vi "HOST_feedback+datapass_accum_8-21-23.vi"() -> ()   [LabVIEW 2020]
uses:
  <vilib>/rvi/interface/nirviMethod/nirviMethod.xnode
  <vilib>/rvi/errors/niLvFpgaMergeErrorWithErrorCode.vi
  <instrlib>/_niInstr/Streaming/v1/Host/niInstr Streaming v1 Host.lvlib
  <vilib>/rvi/interface/nirviReadWriteControl/nirviReadWriteControl.xnode
  <vilib>/rvi/interface/nirviCloseFPGA/nirviCloseFPGA.xnode
  <vilib>/rvi/interface/nirviOpenFPGA/nirviOpenFPGA.xnode
  <vilib>/rvi/interface/Simulation/niFpgaSimulationCallBeginRW.vi
  <vilib>/rvi/errors/niLvFpgaAdjustHostInterfaceError.vi
  NiFpgaLv.dll
  <vilib>/Utility/error.llb/Error Cluster From Error Code.vi
  <vilib>/Utility/file.llb/Write Delimited Spreadsheet (string).vi
  <instrlib>/_niInstr/Streaming/v1/Host/Public/Start Finite Stream.vi
  <instrlib>/_niInstr/Streaming/v1/Host/Public/Wait for Stream.vi
  <instrlib>/_niInstr/Streaming/v1/Host/Public/Start Continuous Stream.vi
  <vilib>/FPGAPlugInAG/Dynamic/niLvFpga_ConfigureFifo_Dynamic.vi
  <vilib>/FPGAPlugInAG/Dynamic/niLvFpga_StartFifo_Dynamic.vi
  <vilib>/FPGAPlugInAG/Dynamic/niLvFpga_ReadFifo_Dynamic.vi
  <vilib>/FPGAPlugInAG/Dynamic/niLvFpga_WriteFifo_Dynamic.vi
  <vilib>/FPGAPlugInAG/Dynamic/niLvFpga_Close_Dynamic.vi
  FPGA Bitfiles/rfsignal_FPGATarget_feedback+datapas_M+I99ZCAYuY.lvbitx
  <vilib>/FPGAPlugInAG/PXIe-7972R/niLvFpga_Open_PXIe-7972R.vi
  <vilib>/rvi/interface/common/dynamic/niFpgaDynamicAddResources.vi
  <vilib>/userdefined/Silver/nirio_resource_slv.ctl
  Controls/Clock Select.ctl
  PID/Typedef/niFpgaPID_ManualControl.ctl
  PID/Typedef/niFpgaPID_PIDGains.ctl
  PID/Typedef/niFpgaPID_OutputRange.ctl
  PID/Typedef/niFpgaPID_SetpointWeightings.ctl
  PID/Typedef/niFpgaPID_PIDActions.ctl
panel:
  in  "Data transfer method":bool
  in  "Downsample":i16
  in  "Signal Delay (us)":i32=5
  out "actions":T1
  out "error":sgl
  out "output":sgl
  out "error 2":sgl
  out "error 3":sgl
  out "output 3":sgl
  out "actions 3":T1
  out "output 2":sgl
  out "actions 2":T1
  in  "Gains Z":T2[](array[typedef]) {"filter coefficient" min=0 max=1; "proportional gain" step=0.125}
  in  "setpoint weighting 3":T3={"proportional weighting (1)"=1.0, "derivative weighting (0)"=0.0} {"derivative weighting (0)" min=0 max=1; "proportional weighting (1)" min=0 max=1}
  in  "output range 3":T4={"output high (Inf)"=inf, "output low (-Inf)"=-inf}
  in  "manual control 3":T5
  in  "reset? (F) 3":bool
  in  "setpoint weighting 2":T3={"proportional weighting (1)"=1.0, "derivative weighting (0)"=0.0} {"derivative weighting (0)" min=0 max=1; "proportional weighting (1)" min=0 max=1}
  in  "output range 2":T4={"output high (Inf)"=inf, "output low (-Inf)"=-inf}
  in  "gains 2":T2 {"filter coefficient" min=0 max=1; "proportional gain" step=0.125}
  in  "manual control 2":T5
  in  "reset? (F) 2":bool
  in  "Feedback scaling z":fxp<+,16,4>
  in  "Feedback scaling x/y":fxp<+,16,4>
  in  "Apply feedback":bool
  in  "Data Trigger Level (V)":dbl
  in  "Record Size":u32=1024
  out "AI":waveform(dbl)[](graph)
  in  "Data Trigger When":enum8{"Trigger Above", "Trigger Below"}(ring)
  in  "Trigger Type":enum8{"Immediate", "Data Trigger", "TRIG input"}(ring)
  in  "Direction switch":bool
  in  "Step gain values":dbl
  in  "?":bool
  in  "% of max CH 1":dbl=85.0
  in  "% of max CH 0":dbl=85.0
  in  "setpoint weighting":T3={"proportional weighting (1)"=1.0, "derivative weighting (0)"=0.0} {"derivative weighting (0)" min=0 max=1; "proportional weighting (1)" min=0 max=1}
  in  "output range":T4={"output high (Inf)"=inf, "output low (-Inf)"=-inf}
  in  "gains":T2 {"filter coefficient" min=0 max=1; "proportional gain" step=0.125}
  in  "manual control":T5
  in  "reset? (F)":bool
  in  "write time ch0":bool
  in  "Record time for power sweep CH0":bool
  in  "Record time for power sweep CH1":bool
  in  "write time ch1":bool
  in  "save path for power calibration (dialog if empty)":path
  out "time check":u16=16
  in  "Cycles per step":u16=30
  in  "Gain Scan Endpoint (CH1)":dbl[](array[numeric])=[100.0, 100.0, 100.0, 100.0, 100.0, 100.0, 100.0, 100.0, 100.0, 100.0, 100.0, 100.0, 100.0, 100.0, 100.0, 100.0, 100.0, 100.0, 100.0, 100.0, 100.0, 100.0, 100.0, 100.0, 100.0, 100.0, 100.0, 100.0, 100.0, 100.0, 100.0, 100.0, 100.0, 100.0, 100.0, 100.0]
  in  "Gain Scan Endpoint (CH0)":dbl[](array[numeric])=[100.0, 100.0, 100.0, 100.0, 100.0, 100.0, 100.0, 100.0, 100.0, 100.0, 100.0, 100.0, 100.0, 100.0, 100.0, 100.0, 100.0, 100.0, 100.0, 100.0, 100.0, 100.0, 100.0, 100.0, 100.0, 100.0, 100.0, 100.0, 100.0, 100.0, 100.0, 100.0, 100.0, 100.0, 100.0, 100.0]
  in  "Scan End Setpoint (CH1)":dbl[](array[numeric])=[23.0, 24.0, 25.0, 26.0, 27.0, 28.0, 23.0, 24.0, 25.0, 26.0, 27.0, 28.0, 23.0, 24.0, 25.0, 26.0, 27.0, 28.0, 23.0, 24.0, 25.0, 26.0, 27.0, 28.0, 23.0, 24.0, 25.0, 26.0, 27.0, 28.0, 23.0, 24.0, 25.0, 26.0, 27.0, 28.0] format="%#_10f"
  in  "Scan CH1":bool
  in  "Scan CH0":bool
  in  "Fq Scan Endpoint (CH0)":dbl[](array[numeric])=[23.0, 23.0, 23.0, 23.0, 23.0, 23.0, 24.0, 24.0, 24.0, 24.0, 24.0, 24.0, 25.0, 25.0, 25.0, 25.0, 25.0, 25.0, 26.0, 26.0, 26.0, 26.0, 26.0, 26.0, 27.0, 27.0, 27.0, 27.0, 27.0, 27.0, 28.0, 28.0, 28.0, 28.0, 28.0, 28.0] format="%#_10f"
  in  "Amp mod on/off":bool[](array[boolean])=[FALSE, FALSE, FALSE, FALSE, FALSE, FALSE, FALSE, FALSE, FALSE]
  in  "Mod Amp (%)":fxp<+,16,1>[](array[numeric])=[1.0, 1.0, 1.0, 1.0, 1.0, 1.0, 1.0, 1.0, 1.0]
  in  "Mod Fq (Hz) 3":dbl[](array[numeric])=[1.0, 1.0, 1.0, 1.0, 1.0, 1.0, 1.0, 1.0, 1.0] format="%#5.5f"
  in  "Wave 2 mod on/off":bool[](array[boolean])=[FALSE, FALSE, FALSE, FALSE, FALSE, FALSE, FALSE, FALSE, FALSE]
  in  "Mod strength (Hz) 2":dbl[](array[numeric])=[100000.0, 100000.0, 100000.0, 100000.0, 100000.0, 100000.0, 100000.0, 100000.0, 100000.0] format="%#_6p"
  in  "Mod Fq (Hz) 2":dbl[](array[numeric])=[1.0, 1.0, 1.0, 1.0, 1.0, 1.0, 1.0, 1.0, 1.0] format="%#5.5f"
  in  "Wave 1 mod on/off":bool[](array[boolean])=[FALSE, FALSE, FALSE, FALSE, FALSE, FALSE, FALSE, FALSE, FALSE]
  in  "Mod strength (Hz)":dbl[](array[numeric])=[100000.0, 100000.0, 100000.0, 100000.0, 100000.0, 100000.0, 100000.0, 100000.0, 100000.0] format="%#_6p"
  in  "Mod Time (Hz)":dbl[](array[numeric])=[1.0, 1.0, 1.0, 1.0, 1.0, 1.0, 1.0, 1.0, 1.0] format="%#5.5p"
  in  "Gain Scan Step Size % (CH1)":dbl=1.0
  in  "Gain Scan Step Size % (CH0)":dbl=1.0
  in  "Fq Scan Step Size MHz (CH1)":dbl=0.1
  in  "Fq Scan Step Size MHz (CH0)":dbl=0.1
  in  "Input pass through\nmode":enum16{"Wire", "Accum-edge"}(ring)
  in  "# of beams":i8=36
  in  "Wave Reader CH 1 (MHz)":dbl[](array[numeric])=[23.0, 24.0, 25.0, 26.0, 27.0, 28.0, 23.0, 24.0, 25.0, 26.0, 27.0, 28.0, 23.0, 24.0, 25.0, 26.0, 27.0, 28.0, 23.0, 24.0, 25.0, 26.0, 27.0, 28.0, 23.0, 24.0, 25.0, 26.0, 27.0, 28.0, 23.0, 24.0, 25.0, 26.0, 27.0, 28.0] format="%#_15f"
  in  "Gain CH 1 (%)":dbl[](array[numeric])=[100.0, 100.0, 100.0, 100.0, 100.0, 100.0, 100.0, 100.0, 100.0, 100.0, 100.0, 100.0, 100.0, 100.0, 100.0, 100.0, 100.0, 100.0, 100.0, 100.0, 100.0, 100.0, 100.0, 100.0, 100.0, 100.0, 100.0, 100.0, 100.0, 100.0, 100.0, 100.0, 100.0, 100.0, 100.0, 100.0]
  in  "Remove transition edges":i32=5
  in  "Time per beam in us":i32=20
  in  "stop":bool
  in  "Gain CH 0 (%)":dbl[](array[numeric])=[100.0, 100.0, 100.0, 100.0, 100.0, 100.0, 100.0, 100.0, 100.0, 100.0, 100.0, 100.0, 100.0, 100.0, 100.0, 100.0, 100.0, 100.0, 100.0, 100.0, 100.0, 100.0, 100.0, 100.0, 100.0, 100.0, 100.0, 100.0, 100.0, 100.0, 100.0, 100.0, 100.0, 100.0, 100.0, 100.0]
  in  "Wave Reader CH 0 (MHz)":dbl[](array[numeric])=[23.0, 23.0, 23.0, 23.0, 23.0, 23.0, 24.0, 24.0, 24.0, 24.0, 24.0, 24.0, 25.0, 25.0, 25.0, 25.0, 25.0, 25.0, 26.0, 26.0, 26.0, 26.0, 26.0, 26.0, 27.0, 27.0, 27.0, 27.0, 27.0, 27.0, 28.0, 28.0, 28.0, 28.0, 28.0, 28.0] format="%#_13f"
  in  "Magnitude Initialization Vpp":dbl[](array[numeric])=[1.0, 1.0] format="%0.2p"
  in  "Frequencies (Hz)":dbl[](array[numeric])=[10000.0, 10000.0] format="%5.0p"
  in  "Signal Type":T6(ring)
  in  "Sampling Info":cluster{"Fs":dbl, "#s":dbl}={"Fs"=163840000.0, "#s"=65536.0} {"Fs" format="%#_5p"}
  out "Error Out":errorcluster
  in  "Update Waveform":bool
  in  "Clock Select":T7 items=["Internal Clock", "Internal Clock w/ Ref via CLK/REF IN", "Internal Clock w/ Ref via Sync Clock", "External Clock via CLK/REF IN"]
  in  "Rate of External Sample Clock (MHz)":u16=100 min=60 max=100 step=1
  in  "RIO Resource":T8="RIO0"
  # "General Feedback Settings"
  # "Time cycle loop processing"
  # "Shared Feedback Controls"
  # "up to 65535"
  # "Don't change"
  # "Waveform Initialization"
  # "Modulation disabled for now while testing FPGA code, too high compiling time for quick turn around"
  # "Controls the Output of the FPGA\nEach row corresponds to one beam created by the AOD\nCH 0 is Output 0 on the FPGA card and controls the () direction on the AOD; CH 1 is Output 1 on the FPGA card and controls the () direction on the AOD\n\nThe  set frequency is the output of the FPGA, this is then mixed with a 50MHz LO to be in the AOD's bandwidth of 75 +- 15MHz\n\nThe gain is the percentage of the 1Vpp initialized voltage to output. It is in percentage and goes from 0 - 100\n\nIt will play the first n rows of tones, \nwhere n is the \"# of beams\" value."
  # "DO NOT CHANGE"
  # "X Feedback"
  # "These allow you to smoothly ramp between frequencies or gain settings for each individual beam.\nThe channels scan independently, but it will simultaneously ramp every fq/gain in the channel to their desired point.\nThey should update to match the main control setting when scanning is not enabled."
  # "Ch 0 Wave Sin Modulation"
  # "Ch 1 Wave Sin Modulation"
  # "Amplitude Sin Modulation"
  # "Do not change these values while waiting for scan"
  # "Main control for the tones played on FPGA analog out 0\nSets the base, static frequency to play"
  # "Main control for the tones played on FPGA analog out 1\nSets the base, static frequency to play"
  # "Ch 0 Output Waveforms"
  # "Ch 1 Output Waveforms"
  # "Y Feedback"
  # "Ch0"
  # "Ch1"
  # "Modulates the output frequencies of CH 0 in a sine wave pattern\n\nMod time: Sets how fast the modulation goes\n     (e.g. 1 Hz means it will go through a full cycle in 1 second)\n\nMod strength: Sets the amplitude of the modulation\n     (e.g. 100kHz means that the frequency will go between \n      set frequency + 100kHz and set frequency - 100kHz)"
  # "Modulates the output frequencies of CH 1 in a sine wave pattern\n\nMod time: Sets how fast the modulation goes\n     (e.g. 1 Hz means it will go through a full cycle in 1 second)\n\nMod strength: Sets the amplitude of the modulation\n     (e.g. 100kHz means that the frequency will go between \n      set frequency + 100kHz and set frequency - 100kHz)"
  # "Modulates the output amplitude of CH 0 in a sine wave pattern\n\nMod time: Sets how fast the modulation goes\n     (e.g. 1 Hz means it will go through a full cycle in 1 second)\n\nMod strength: Sets the amplitude of the modulation\n     (e.g. 5% means that the amplitude will go between \n      set amp + 5%  and set amp  - 5%)"
  # "Z\nFeedback"
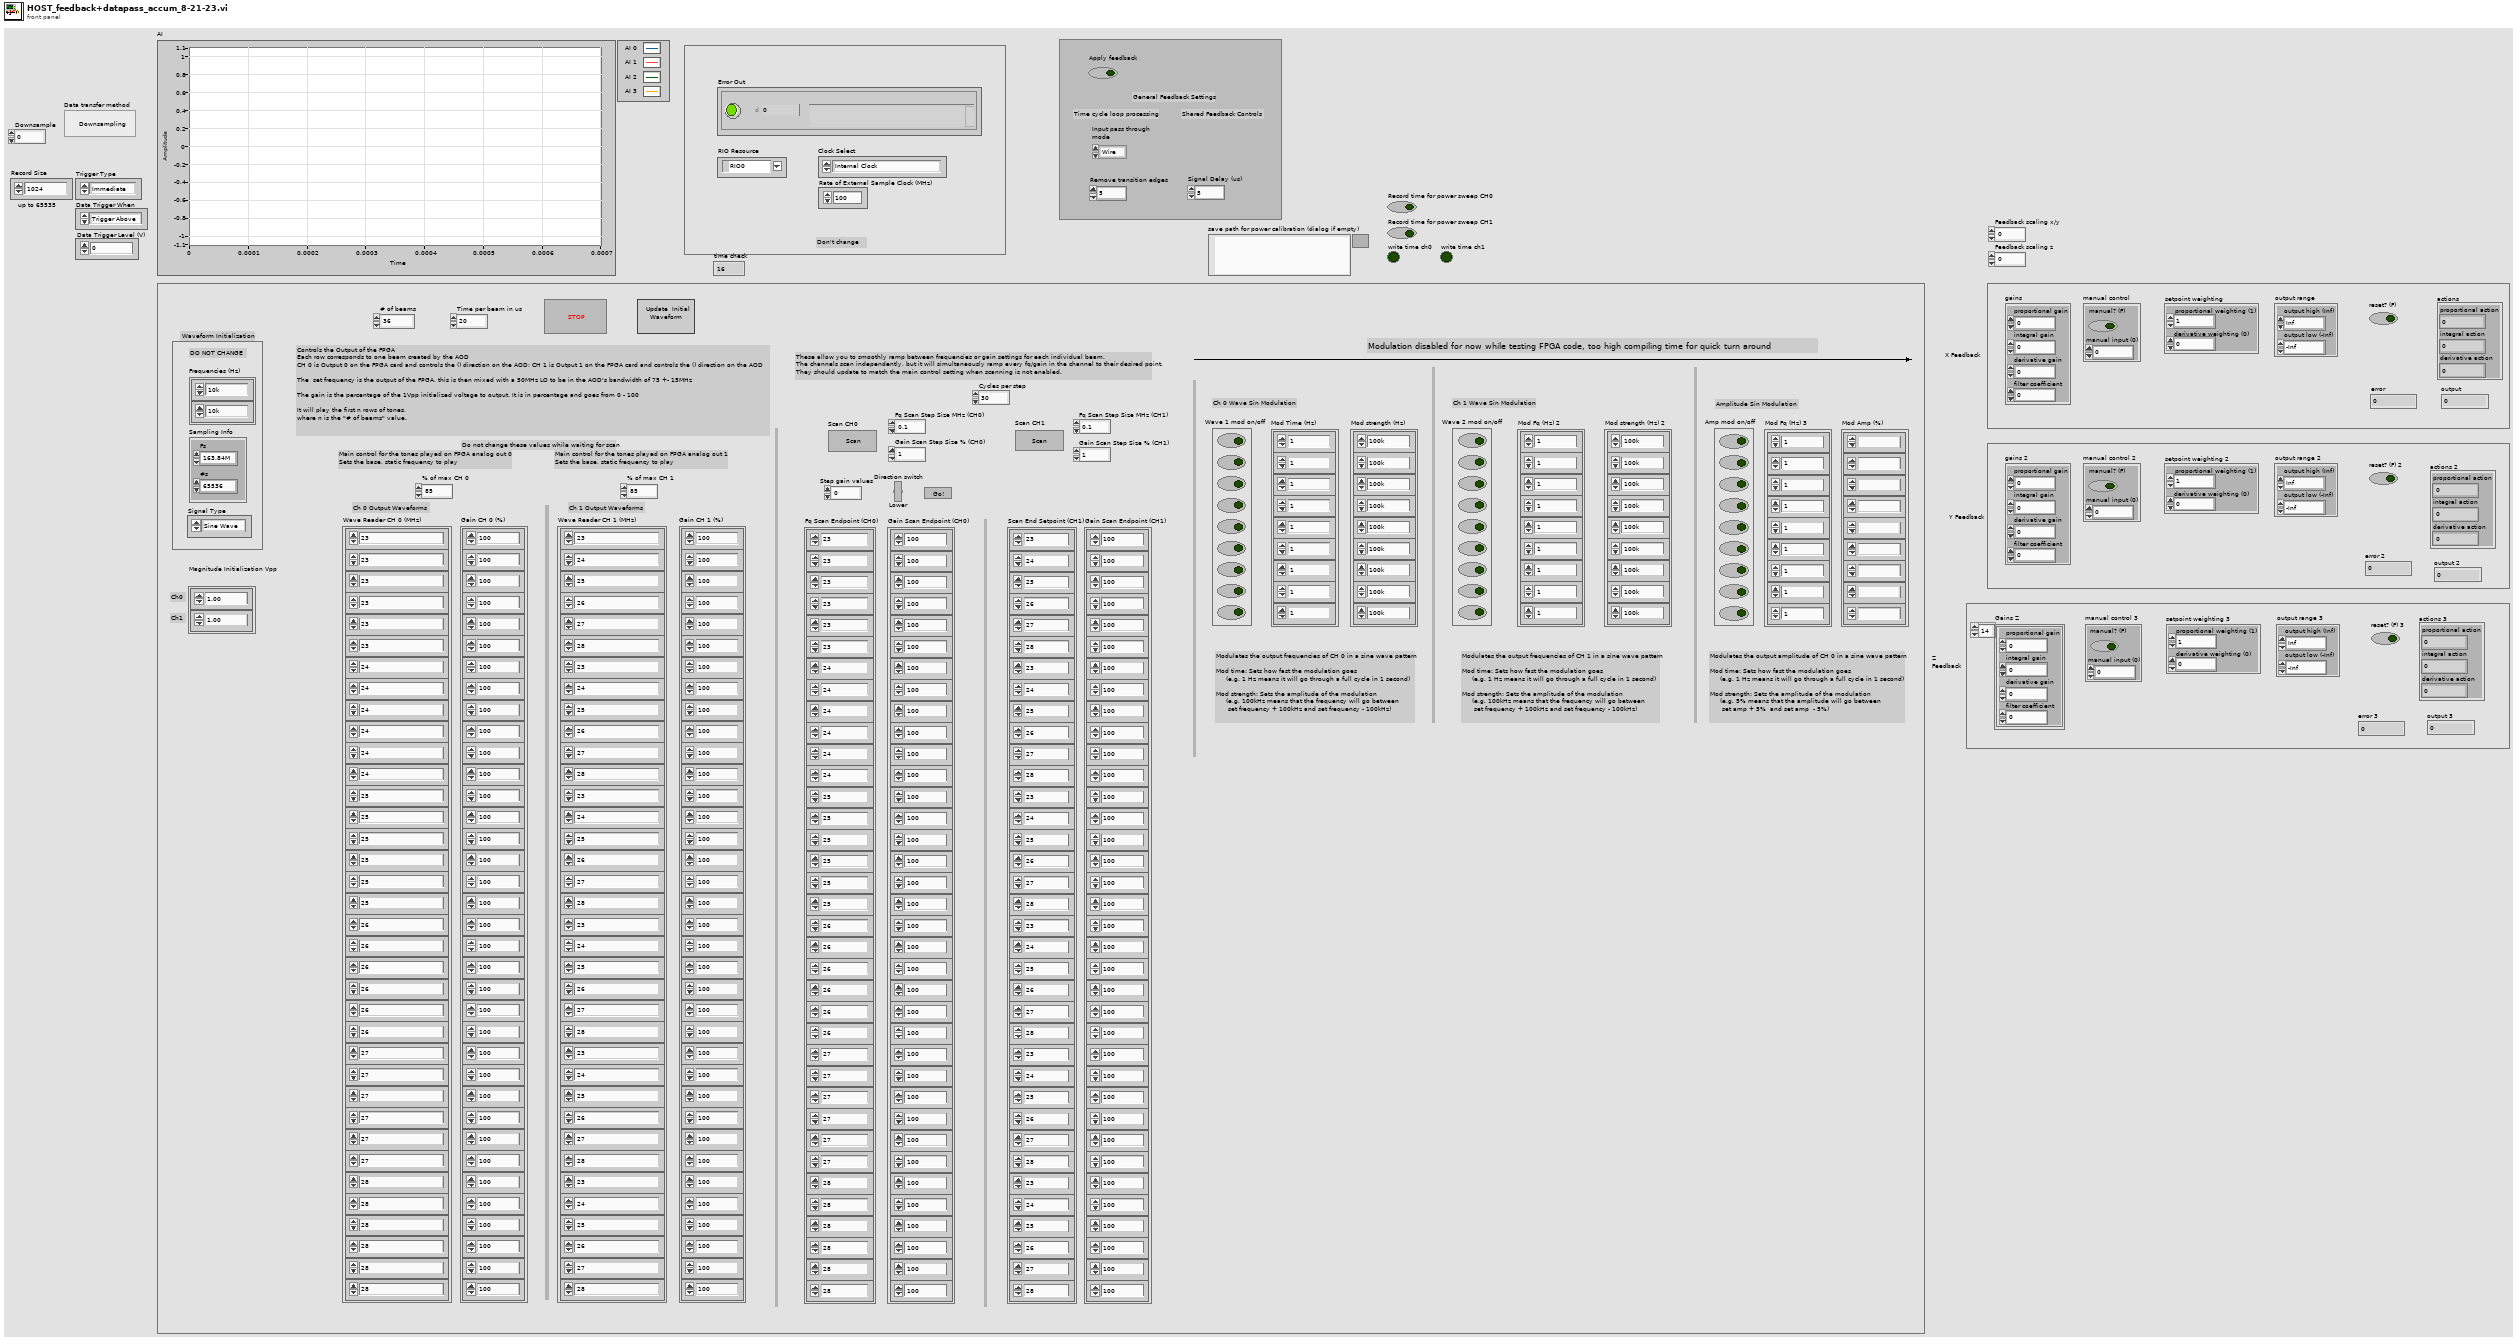
[diagram p1: front panel]
types:
  T1 = typedef "niFpgaPID_PIDActions.ctl" = cluster{"proportional action":sgl, "integral action":sgl, "derivative action":sgl}
  T2 = typedef "niFpgaPID_PIDGains.ctl" = cluster{"proportional gain":sgl, "integral gain":sgl, "derivative gain":sgl, "filter coefficient":sgl}
  T3 = typedef "niFpgaPID_SetpointWeightings.ctl" = cluster{"proportional weighting (1)":sgl, "derivative weighting (0)":sgl}
  T4 = typedef "niFpgaPID_OutputRange.ctl" = cluster{"output high (Inf)":sgl, "output low (-Inf)":sgl}
  T5 = typedef "niFpgaPID_ManualControl.ctl" = cluster{"manual? (F)":bool, "manual input (0)":sgl}
  T6 = enum16{"Sine Wave", "Triangle Wave", "Square Wave", "Sawtooth Wave"}
  T7 = typedef "Clock Select.ctl" = u16
  T8 = typedef "nirio_resource_slv.ctl" = tag
  T9 = cluster{"proportional action":sgl, "integral action":sgl, "derivative action":sgl}
  T10 = cluster{"level":i16, "trigger when":enum8{"Trigger Above", "Trigger Below"}}
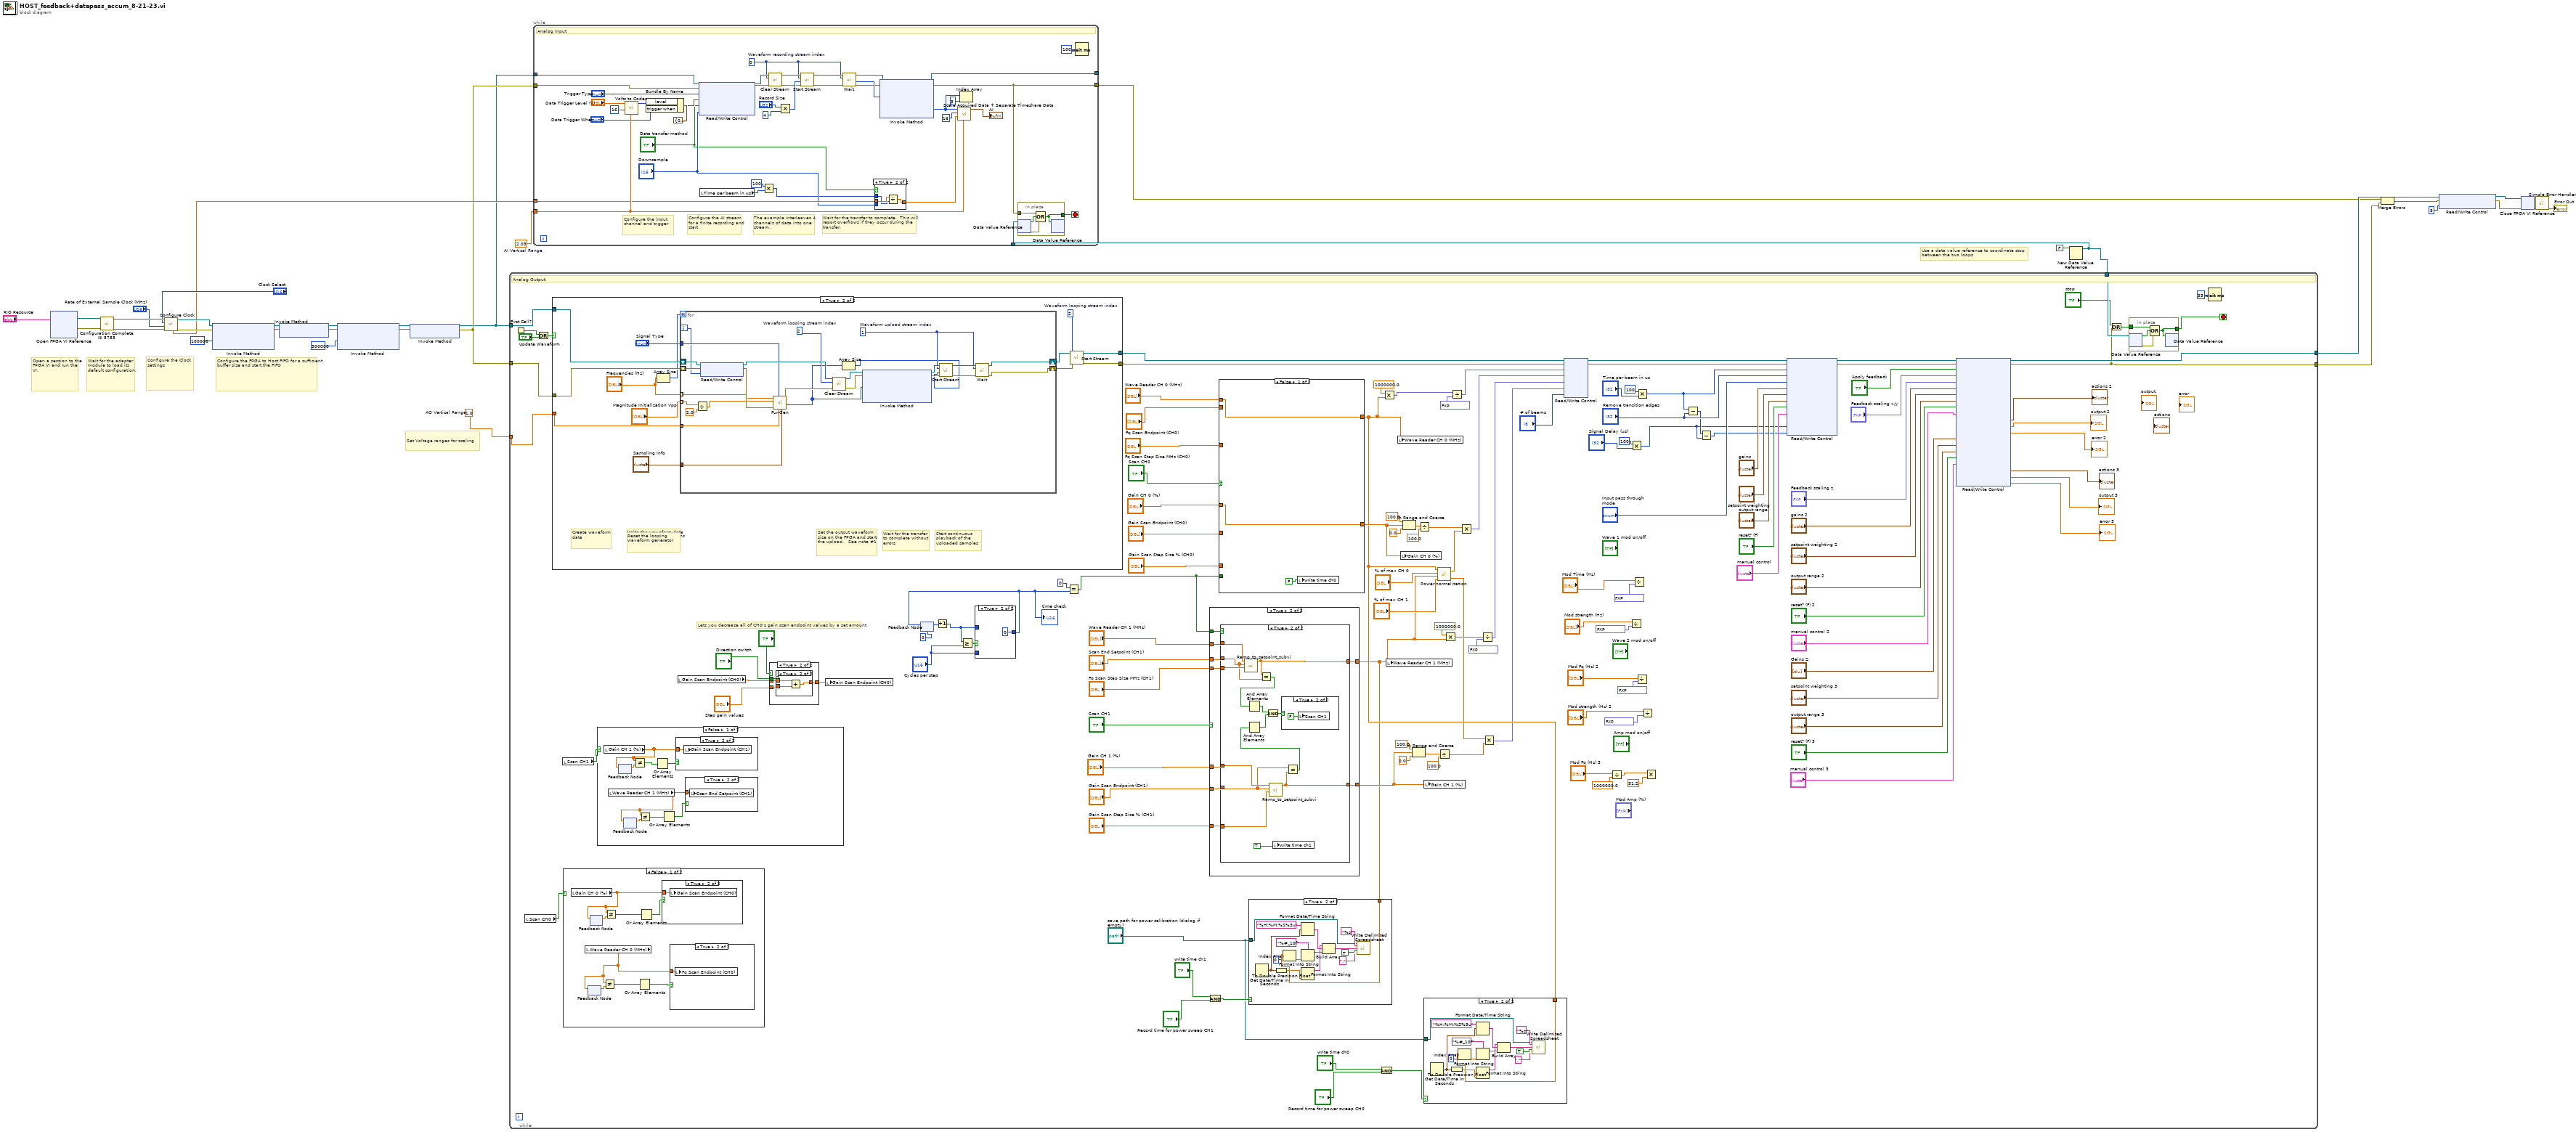
[diagram p0: block diagram]
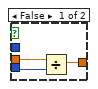
[diagram p2: hidden frame]
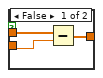
[diagram p4: hidden frame]
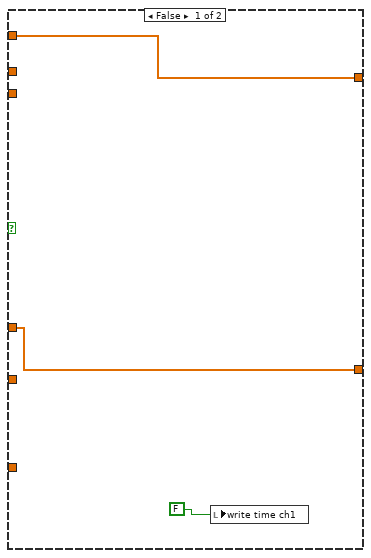
[diagram p7: hidden frame]
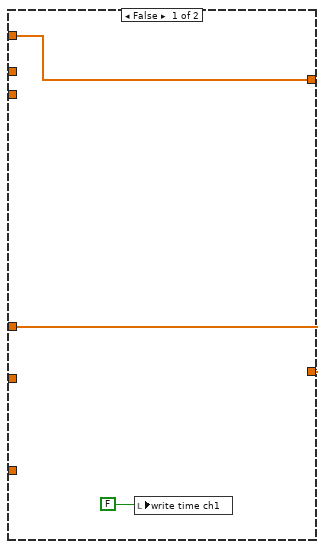
[diagram p8: hidden frame]
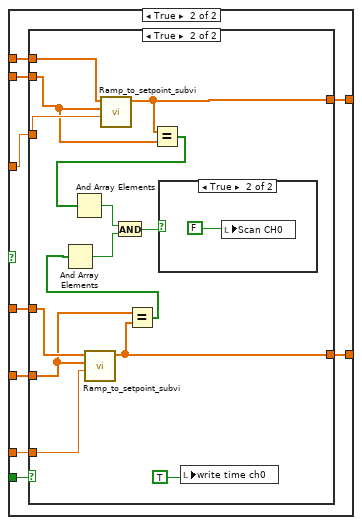
[diagram p10: hidden frame]
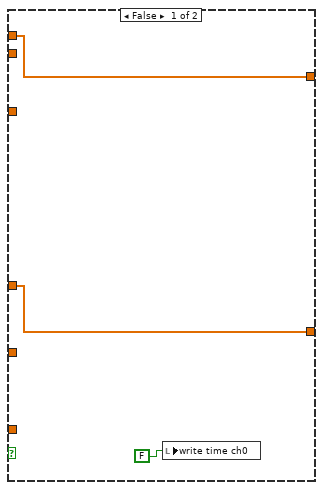
[diagram p11: hidden frame]
diagram:
  w13 = 2.03  # AI Vertical Range
  w21 = 1.0  # AO Vertical Range
  # "Use a data value reference to coordinate stop between the two loops"
  # "Set Voltage ranges for scaling"
  # "Configure the Clock settings"
  # "Configure the FPGA to Host FIFO for a sufficient buffer size and start the FIFO"
  # "Wait for the adapter module to load its default configuration."
  # "Open a session to the FPGA VI and run the VI."
  n1 = xnode "Open FPGA VI Reference"("resource name"="RIO Resource") -> ("FPGA VI Reference Out"=w19:refnum<k20>, "error out"=w18:errorcluster)  [unwired: 1 in]
  n2 = call "Configuration Complete NI 5783.vi"("error in"=w18, "FPGA VI Reference In"=w19) -> ("error out"=w29:errorcluster, "FPGA VI Reference Out"=w30:refnum<k20>)  [unwired: 7 in, 1 out]
  n3 = call "Configure Clock.vi"("error in (no error)"=w29, "Rate of External Sample Clock (MHz)"="Rate of External Sample Clock (MHz)", "Clock Select"="Clock Select", "FPGA VI Reference In"=w30) -> ("error out"=w27:errorcluster, "FPGA VI Reference Out"=w28:refnum<k20>, "Sampling Rate"=w12:dbl)  [unwired: 3 in, 2 out]
  n4 = xnode "Invoke Method"("FPGA VI Reference In"=w28, "error in"=w27, "Requested Depth"=u32 100000) -> ("FPGA VI Reference Out"=w33:refnum<k20>, "error out"=w32:errorcluster)  [unwired: 1 out]
  n5 = xnode "Invoke Method"("FPGA VI Reference In"=w33, "error in"=w32) -> ("FPGA VI Reference Out"=w4:refnum<k20>, "error out"=w7:errorcluster)
  n6 = xnode "Invoke Method"("FPGA VI Reference In"=w4, "error in"=w7, "Requested Depth"=u32 300000) -> ("FPGA VI Reference Out"=w3:refnum<k20>, "error out"=w6:errorcluster)  [unwired: 1 out]
  n7 = xnode "Invoke Method"("FPGA VI Reference In"=w3, "error in"=w6) -> ("FPGA VI Reference Out"=w2:refnum<k20>, "error out"=w5:errorcluster)
  n8 = New Data Value Reference(data value=FALSE ("Stopped")) -> (data value reference=w10:refnum<data-value>)  [unwired: 1 in, 1 out]
  n9 = while {
    tunnel: w5 -> [w157]
    tunnel: w2 -> [w163]
    tunnel: [w61] -> w17
    tunnel: w10 -> [w158]
    tunnel: w21 -> [w156]
    tunnel: [w59] -> w8
    stop <- w66 stop-if-true
    # "Lets you decrease all of CH0's gain scan endpoint values by a set amount"
    # "Analog Output"
    n10 = First Call?() -> (First Call?: T/F=w159:bool)
    n11 = local read "Scan CH0"() -> (w109:bool)
    n12 = Or(x=w159, y="Update Waveform") -> (x .or. y?=w160:bool)
    n13 = case shown="True" w160 {
      tunnel: [w292 w305] -> w155
      tunnel: [w291 w304] -> w154
      tunnel: w163 -> [w292 w302]
      tunnel: w157 -> [w291 w301]
      tunnel: w156 -> [_ w303]
      frame False {
      }
      frame True {
        w300 = 2  # Waveform looping stream index
        # "Loop over the waveforms to combine"
        # "Reset the looping waveform generator"
        # "Start continuous playback of the uploaded samples"
        # "Wait for the transfer to complete without errors"
        # "Set the output waveform size on the FPGA and start the upload.   See note #1"
        # "Write the waveform data to the FPGA for generation"
        # "Create waveform data"
        n14 = Array Size(array="Frequencies (Hz)") -> (size(s)=w295:i32)
        n15 = for {
          N: w295 -> [_]
          tunnel: w303 -> [w320]
          shift-right: [w314] -> w299
          shift-left: w302 -> [w319]
          shift-right: [w313] -> w298
          shift-left: w301 -> [w317]
          tunnel: "Frequencies (Hz)" -> [w312] mode=indexing
          tunnel: "Magnitude Initialization Vpp" -> [w308] mode=indexing
          tunnel: "Sampling Info" -> [w311]
          tunnel: "Signal Type" -> [w310]
          i -> [w309]
          w321 = 2  # Waveform looping stream index
          w326 = 1  # Waveform upload stream index
          n16 = Divide(x=w308, y=2.0) -> (x/y=w307:dbl)
          n17 = xnode "Read/Write Control"("FPGA VI Reference In"=w319, "error in"=w317, "Upload selector"=w309) -> ("FPGA VI Reference Out"=w318:refnum<k20>, "error out"=w316:errorcluster)
          n18 = call "FunGen.vi"("sampling info"=w311, "range (Vpp)"=w320, "signal type"=w310, "error in (no error)"=w316, "amplitude"=w307, "frequency"=w312) -> ("error out"=w322:errorcluster, "Waveform Data"=w315:i16[])  [unwired: 2 in, 2 out]
          n19 = call <instrlib>:"Clear Stream.vi"("error in (no error)"=w322, "stream index"=w321, "refnum in"=w318) -> ("error out"=w324:errorcluster, "refnum out"=w325:refnum<k20>)  [unwired: 7 in]
          n20 = Array Size(array=w315) -> (size(s)=w323:i32)
          n21 = xnode "Invoke Method"("FPGA VI Reference In"=w325, "error in"=w324, "Data"=w315) -> ("FPGA VI Reference Out"=w330:refnum<k20>, "error out"=w329:errorcluster)  [unwired: 1 in, 1 out]
          n22 = call-poly <instrlib>:"Start Stream.vi"("error in (no error)"=w329, "num samples"=w323, "stream index"=w326, "refnum in"=w330) -> ("error out"=w327:errorcluster, "refnum out"=w328:refnum<k20>)  [unwired: 6 in]
          n23 = call-poly <instrlib>:"Wait.vi"("error in (no error)"=w327, "stream index"=w326, "refnum in"=w328) -> ("error out"=w313:errorcluster, "refnum out"=w314:refnum<k20>)  [unwired: 5 in, 2 out]
        }
        n24 = call-poly <instrlib>:"Start Stream.vi"("error in (no error)"=w298, "stream index"=w300, "refnum in"=w299) -> ("error out"=w304:errorcluster, "refnum out"=w305:refnum<k20>)  [unwired: 7 in]
      }
    }
    n25 = local read "Scan CH1"() -> (w110:bool)
    n26 = case shown="False" w109 {
      frame False {
        n27 = local read "Gain CH 0 (%)"() -> (w267:dbl[])
        n28 = local read "Wave Reader CH 0 (MHz)"() -> (w274:dbl[])
        n29 = feedback-in #1(w274) -> ()
        n30 = feedback #1() -> (w273:dbl[])  [unwired: 1 in]
        n31 = feedback #2() -> (w270:dbl[])  [unwired: 1 in]
        n32 = feedback-in #2(w267) -> ()
        n33 = Not Equal?(x=w274, y=w273) -> (x != y?=w272:bool[])
        n34 = Not Equal?(x=w267, y=w270) -> (x != y?=w269:bool[])
        n35 = Or Array Elements(Boolean array=w272) -> (logical OR=w271:bool)
        n36 = Or Array Elements(Boolean array=w269) -> (logical OR=w268:bool)
        n37 = case shown="True" w268 {
          tunnel: w267 -> [_ w275]
          frame False {
          }
          frame True {
            n38 = local write "Gain Scan Endpoint (CH0)"(w275) -> ()
          }
        }
        n39 = case shown="True" w271 {
          tunnel: w274 -> [_ w276]
          frame False {
          }
          frame True {
            n40 = local write "Fq Scan Endpoint (CH0)"(w276) -> ()
          }
        }
      }
      frame True {
      }
    }
    n41 = case shown="False" w110 {
      frame False {
        n42 = local read "Gain CH 1 (%)"() -> (w277:dbl[])
        n43 = local read "Wave Reader CH 1 (MHz)"() -> (w281:dbl[])
        n44 = feedback #3() -> (w280:dbl[])  [unwired: 1 in]
        n45 = feedback-in #3(w277) -> ()
        n46 = feedback #4() -> (w284:dbl[])  [unwired: 1 in]
        n47 = feedback-in #4(w281) -> ()
        n48 = Not Equal?(x=w277, y=w280) -> (x != y?=w279:bool[])
        n49 = Not Equal?(x=w281, y=w284) -> (x != y?=w283:bool[])
        n50 = Or Array Elements(Boolean array=w279) -> (logical OR=w278:bool)
        n51 = Or Array Elements(Boolean array=w283) -> (logical OR=w282:bool)
        n52 = case shown="True" w278 {
          tunnel: w277 -> [_ w285]
          frame False {
          }
          frame True {
            n53 = local write "Gain Scan Endpoint (CH1)"(w285) -> ()
          }
        }
        n54 = case shown="True" w282 {
          tunnel: w281 -> [_ w286]
          frame False {
          }
          frame True {
            n55 = local write "Scan End Setpoint (CH1)"(w286) -> ()
          }
        }
      }
      frame True {
      }
    }
    n56 = local read "Gain Scan Endpoint (CH0)"() -> (w68:dbl[])
    n57 = case shown="True" "?" {
      tunnel: w68 -> [w164 w167]
      tunnel: [w164 w168] -> w69
      tunnel: "Step gain values" -> [_ w166]
      tunnel: "Direction switch" -> [_ w165]
      frame False {
      }
      frame True {
        n58 = case shown="True" w165 {
          tunnel: [w171 w173] -> w168
          tunnel: w167 -> [w170 w172]
          tunnel: w166 -> [w169 w174]
          frame False {
            n59 = Subtract(x=w170, y=w169) -> (x-y=w171:dbl[])
          }
          frame True {
            n60 = Add(x=w172, y=w174) -> (x+y=w173:dbl[])
          }
        }
      }
    }
    n61 = local write "Gain Scan Endpoint (CH0)"(w69) -> ()
    n62 = feedback #5(u16 0) -> (w105:u16)
    n63 = Increment(x=w105) -> (x+1=w103:u16)
    n64 = Greater Or Equal?(x=w103, y="Cycles per step") -> (x >= y?=w104:bool)
    n65 = case shown="True" w104 {
      tunnel: w103 -> [w265 _]
      tunnel: "Cycles per step" -> [_ _]
      tunnel: [w265 u16 0] -> w98
      frame False {
      }
      frame True {
      }
    }
    "time check" <- w98
    n66 = feedback-in #5(w98) -> ()
    n67 = Equal?(x=u16 0, y=w98) -> (x = y?=w99:bool)
    n68 = And(x="write time ch1", y="Record time for power sweep CH1") -> (x .and. y?=w97:bool)
    n69 = case shown="True" "Scan CH1" {
      tunnel: "Fq Scan Step Size MHz (CH1)" -> [_ w216]
      tunnel: [w207 w215] -> w77
      tunnel: "Wave Reader CH 1 (MHz)" -> [w207 w214]
      tunnel: "Scan End Setpoint (CH1)" -> [_ w213]
      tunnel: "Gain Scan Step Size % (CH1)" -> [_ w212]
      tunnel: "Gain CH 1 (%)" -> [w206 w211]
      tunnel: "Gain Scan Endpoint (CH1)" -> [_ w210]
      tunnel: [w206 w209] -> w111
      tunnel: w99 -> [_ w208]
      frame False {
        n70 = local write "write time ch1"(FALSE) -> ()
      }
      frame True {
        n71 = case shown="True" w208 {
          tunnel: w214 -> [w219 w233]
          tunnel: w213 -> [_ w231]
          tunnel: w216 -> [_ w232]
          tunnel: [w219 w230] -> w215
          tunnel: w211 -> [w218 w228]
          tunnel: w210 -> [_ w227]
          tunnel: w212 -> [_ w226]
          tunnel: [w218 w221] -> w209
          frame False {
            n72 = local write "write time ch1"(FALSE) -> ()
          }
          frame True {
            n73 = call "Ramp_to_setpoint_subvi.vi"("Numeric"=w232, "Scan to Fq (CH0)"=w231, "Wave Reader CH 0 (Y)"=w233) -> ("Array"=w230:dbl[])  [unwired: 8 in]
            n74 = Equal?(x=w230, y=w231) -> (x = y?=w229:bool[])
            n75 = And Array Elements(Boolean array=w229) -> (logical AND=w223:bool)
            n76 = call "Ramp_to_setpoint_subvi.vi"("Numeric"=w226, "Scan to Fq (CH0)"=w227, "Wave Reader CH 0 (Y)"=w228) -> ("Array"=w221:dbl[])  [unwired: 8 in]
            n77 = local write "write time ch1"(TRUE) -> ()
            n78 = Equal?(x=w227, y=w221) -> (x = y?=w222:bool[])
            n79 = And Array Elements(Boolean array=w222) -> (logical AND=w224:bool)
            n80 = And(x=w223, y=w224) -> (x .and. y?=w225:bool)
            n81 = case shown="True" w225 {
              frame False {
              }
              frame True {
                n82 = local write "Scan CH1"(FALSE) -> ()
              }
            }
          }
        }
      }
    }
    n83 = case shown="False" "Scan CH0" {
      tunnel: "Fq Scan Step Size MHz (CH0)" -> [_ w246]
      tunnel: "Wave Reader CH 0 (MHz)" -> [w237 w245]
      tunnel: "Fq Scan Endpoint (CH0)" -> [_ w244]
      tunnel: [w237 w243] -> w78
      tunnel: "Gain CH 0 (%)" -> [w236 w242]
      tunnel: "Gain Scan Endpoint (CH0)" -> [_ w241]
      tunnel: [w236 w240] -> w119
      tunnel: "Gain Scan Step Size % (CH0)" -> [_ w239]
      tunnel: w99 -> [_ w238]
      frame False {
        n84 = local write "write time ch0"(FALSE) -> ()
      }
      frame True {
        n85 = case shown="True" w238 {
          tunnel: w245 -> [w249 w263]
          tunnel: w244 -> [_ w261]
          tunnel: w246 -> [_ w262]
          tunnel: [w249 w260] -> w243
          tunnel: w242 -> [w248 w258]
          tunnel: w241 -> [_ w255]
          tunnel: w239 -> [_ w257]
          tunnel: [w248 w256] -> w240
          frame False {
            n86 = local write "write time ch0"(FALSE) -> ()
          }
          frame True {
            n87 = call "Ramp_to_setpoint_subvi.vi"("Numeric"=w257, "Scan to Fq (CH0)"=w255, "Wave Reader CH 0 (Y)"=w258) -> ("Array"=w256:dbl[])  [unwired: 8 in]
            n88 = call "Ramp_to_setpoint_subvi.vi"("Numeric"=w262, "Scan to Fq (CH0)"=w261, "Wave Reader CH 0 (Y)"=w263) -> ("Array"=w260:dbl[])  [unwired: 8 in]
            n89 = Equal?(x=w255, y=w256) -> (x = y?=w254:bool[])
            n90 = And Array Elements(Boolean array=w254) -> (logical AND=w251:bool)
            n91 = Equal?(x=w260, y=w261) -> (x = y?=w259:bool[])
            n92 = And Array Elements(Boolean array=w259) -> (logical AND=w252:bool)
            n93 = And(x=w252, y=w251) -> (x .and. y?=w253:bool)
            n94 = case shown="True" w253 {
              frame False {
              }
              frame True {
                n95 = local write "Scan CH0"(FALSE) -> ()
              }
            }
            n96 = local write "write time ch0"(TRUE) -> ()
          }
        }
      }
    }
    n97 = case shown="True" w97 {
      tunnel: w77 -> [_ w197]
      tunnel: "save path for power calibration (dialog if empty)" -> [_ w190]
      frame False {
      }
      frame True {
        n98 = Get Date/Time In Seconds() -> (seconds since 1Jan1904=w193:timestamp)
        n99 = To Double Precision Float(number=w193) -> (double precision float=w192:dbl)
        n100 = Index Array(array=w197, index=0) -> (element=w195:dbl)
        n101 = Format Date/Time String(time format string (%c)="%H:%M:%S%3u", seconds (now)=w193) -> (date/time string=w200:string)  [unwired: 1 in]
        n102 = Format Into String(format string="%#_10f", w195) -> (resulting string=w199:string)  [unwired: 2 in, 1 out]
        n103 = Format Into String(w192) -> (resulting string=w191:string)  [unwired: 3 in, 1 out]
        n104 = Build Array(w191, w200, w199) -> (w194:string[])
        n105 = call-poly <vilib>:"Write Delimited Spreadsheet.vi"("file path (dialog if empty)"=w190, "format (%s)"="%s" ("format (%.3f)"), "1D data"=w194, "append to file? (new file:F)"=TRUE, "delimiter (\\t)"="," ("delimiter (\\t)")) -> ()  [unwired: 9 in, 2 out]
      }
    }
    n106 = And(x="write time ch0", y="Record time for power sweep CH0") -> (x .and. y?=w93:bool)
    n107 = Multiply(x=1000000.0, y=w78) -> (x*y=w131:fxp<+/-,64,32>[])
    n108 = local write "Wave Reader CH 1 (MHz)"(w77) -> ()
    n109 = local write "Wave Reader CH 0 (MHz)"(w78) -> ()
    n110 = local write "Gain CH 0 (%)"(w119) -> ()
    n111 = In Range and Coerce(upper limit=100.0, x=w119, lower limit=0.0) -> (coerced(x)=w122:dbl[])  [unwired: 1 out]
    n112 = In Range and Coerce(upper limit=100.0, x=w111, lower limit=0.0) -> (coerced(x)=w117:dbl[])  [unwired: 1 out]
    n113 = Divide(x=w122, y=100.0) -> (x/y=w82:dbl[])
    n114 = local write "Gain CH 1 (%)"(w111) -> ()
    n115 = case shown="True" w93 {
      tunnel: w78 -> [_ w182]
      tunnel: "save path for power calibration (dialog if empty)" -> [_ w175]
      frame False {
      }
      frame True {
        n116 = Get Date/Time In Seconds() -> (seconds since 1Jan1904=w178:timestamp)
        n117 = To Double Precision Float(number=w178) -> (double precision float=w177:dbl)
        n118 = Index Array(array=w182, index=0) -> (element=w180:dbl)
        n119 = Format Date/Time String(time format string (%c)="%H:%M:%S%3u", seconds (now)=w178) -> (date/time string=w185:string)  [unwired: 1 in]
        n120 = Format Into String(format string="%#_10f", w180) -> (resulting string=w184:string)  [unwired: 2 in, 1 out]
        n121 = Format Into String(w177) -> (resulting string=w176:string)  [unwired: 3 in, 1 out]
        n122 = Build Array(w176, w185, w184) -> (w179:string[])
        n123 = call-poly <vilib>:"Write Delimited Spreadsheet.vi"("file path (dialog if empty)"=w175, "format (%s)"="%s" ("format (%.3f)"), "1D data"=w179, "append to file? (new file:F)"=TRUE, "delimiter (\\t)"="," ("delimiter (\\t)")) -> ()  [unwired: 9 in, 2 out]
      }
    }
    n124 = call "Power normalization.vi"("% of max CH 1"="% of max CH 1", "CH 1 frequency"=w77, "% of max CH 0"="% of max CH 0", "CH 0 frequency"=w78) -> ("Normalized CH1"=w74:dbl[], "Normalized CH 0"=w79:dbl[])
    n125 = Divide(x=w117, y=100.0) -> (x/y=w75:dbl[])
    n126 = Multiply(x=1000000.0, y=w77) -> (x*y=w128:fxp<+/-,64,32>[])
    n127 = Divide(x=w131, y=fxp<+,32,16> 6103.515625) -> (x/y=w90:fxp<+,33,16>[])
    n128 = Multiply(x=w82, y=w79) -> (x*y=w83:fxp<+,32,4>[])
    n129 = Divide(x=w128, y=fxp<+,32,16> 6103.515625) -> (x/y=w89:fxp<+,33,16>[])
    n130 = Multiply(x=w74, y=w75) -> (x*y=w76:fxp<+,32,4>[])
    n131 = xnode "Read/Write Control"("FPGA VI Reference In"=w155, "error in"=w154, "Wave 1"=w90, "Amp 1"=w83, "Wave 2"=w89, "Amp 2"=w76, "Size"="# of beams") -> ("FPGA VI Reference Out"=w152:refnum<k20>, "error out"=w151:errorcluster)
    n132 = Divide(x="Mod Fq (Hz) 3", y=1000000.0) -> (x/y=w141:dbl[])
    n133 = Divide(x="Mod strength (Hz)", y=fxp<+,32,16> 6103.515625) -> ()  [unwired: 1 out]
    n134 = Multiply(x=100, y="Signal Delay (us)") -> (x*y=w35:i32)
    n135 = Divide(x="Mod Time (Hz)", y=fxp<+,32,16> 6103.515625) -> ()  [unwired: 1 out]
    n136 = Divide(x="Mod Fq (Hz) 2", y=fxp<+,32,16> 6103.515625) -> ()  [unwired: 1 out]
    n137 = Multiply(x=100, y="Time per beam in us") -> (x*y=w38:i32)
    n138 = Divide(x="Mod strength (Hz) 2", y=fxp<+,32,16> 6103.515625) -> ()  [unwired: 1 out]
    n139 = Multiply(x=w141, y=51.2) -> ()  [unwired: 1 out]
    n140 = Subtract(x=w38, y="Remove transition edges") -> (x-y=w36:i32)
    n141 = Subtract(x=w36, y=w35) -> (x-y=w34:i32)
    n142 = xnode "Read/Write Control"("FPGA VI Reference In"=w152, "error in"=w151, "Timeshare"=w38, "Edge size"="Remove transition edges", "Pass selector"="Input pass through\nmode", "gains"="gains", "setpoint weighting"="setpoint weighting", "output range"="output range", "reset? (F)"="reset? (F)", "manual control"="manual control", "Signal Delay"=w35, "Data collection size"=w34) -> ("FPGA VI Reference Out"=w62:refnum<k20>, "error out"=w63:errorcluster)  [unwired: 1 in]
    n143 = xnode "Read/Write Control"("FPGA VI Reference In"=w62, "error in"=w63, "Apply feedback"="Apply feedback", "Feedback scaling x/y"="Feedback scaling x/y", "Feedback scaling z"="Feedback scaling z", "gains 2"="gains 2", "setpoint weighting 2"="setpoint weighting 2", "output range 2"="output range 2", "reset? (F) 2"="reset? (F) 2", "manual control 2"="manual control 2", "Gains Z"="Gains Z", "setpoint weighting 3"="setpoint weighting 3", "output range 3"="output range 3", "reset? (F) 3"="reset? (F) 3", "manual control 3"="manual control 3") -> ("FPGA VI Reference Out"=w61:refnum<k20>, "error out"=w59:errorcluster, "actions 2"=→"actions 2":T9, "output 2"=→"output 2":sgl, "error 2"=→"error 2":sgl, "actions 3"=→"actions 3":T9, "output 3"=→"output 3":sgl, "error 3"=→"error 3":sgl)
    n144 = Or(x="stop", y=w59) -> (x .or. y?=w65:bool)
    n145 = in-place {
      in-place-border: [w289] -> w66
      in-place-border: w65 -> [w287]
      n146 = in-place-dvr #6(w158) -> (w290:bool, w288:errorcluster)
      n147 = Compound Arithmetic op=OR(w287, w290, w288) -> (w289:bool)
      n148 = in-place-dvr #6(w289) -> ()  [unwired: 2 out]
    }
    n149 = Wait (ms)(milliseconds to wait=u32 33) -> ()  [unwired: 1 out]
  }
  n150 = while {
    tunnel: [w368] -> _
    tunnel: w2 -> [w367]
    tunnel: w13 -> [w351]
    tunnel: w10 -> [w364]
    tunnel: w5 -> [w366]
    tunnel: [w355] -> w9
    tunnel: w12 -> [w339]
    stop <- w365 stop-if-true
    w343 = 0  # Waveform recording stream index
    # "The example interleaves 4 channels of data into one stream."
    # "Wait for the transfer to complete.  This will report overflows if they occur during the transfer."
    # "Configure the AI stream for a finite recording and start"
    # "Configure the input channel and trigger"
    # "Analog Input"
    n151 = call "Volts to Codes.vi"("range (Vpp)"=w351, "Number of Bits"=i16 16, "Volts In"="Data Trigger Level (V)") -> ("ADC Codes Out"=w352:i16)  [unwired: 8 in]
    n152 = Bundle By Name(cluster=T10 {"level"=0, "trigger when"=enum."Trigger Above"} ("Trigger Configuration"), "level"=w352, "trigger when"="Data Trigger When") -> (w342:T10)
    n153 = xnode "Read/Write Control"("FPGA VI Reference In"=w367, "error in"=w366, "Trigger Type"="Trigger Type", "Trigger Configuration"=w342, "Data transfer method"="Data transfer method", "Downsample"="Downsample") -> ("FPGA VI Reference Out"=w347:refnum<k20>, "error out"=w346:errorcluster)
    n154 = local read "Time per beam in us"() -> (w334:i32)
    n155 = Multiply(x=100, y=w334) -> (x*y=w333:i32)
    n156 = call <instrlib>:"Clear Stream.vi"("error in (no error)"=w346, "stream index"=w343, "refnum in"=w347) -> ("error out"=w345:errorcluster, "refnum out"=w344:refnum<k20>)  [unwired: 7 in]
    n157 = Multiply(x="Record Size", y=u16 4) -> (x*y=w348:u32)
    n158 = call-poly <instrlib>:"Start Stream.vi"("error in (no error)"=w345, "num samples"=w348, "stream index"=w343, "refnum in"=w344) -> ("error out"=w360:errorcluster, "refnum out"=w358:refnum<k20>)  [unwired: 6 in]
    n159 = call-poly <instrlib>:"Wait.vi"("error in (no error)"=w360, "stream index"=w343, "refnum in"=w358) -> ("error out"=w356:errorcluster, "samples transferred"=w359:u64, "refnum out"=w357:refnum<k20>)  [unwired: 5 in, 1 out]
    n160 = case shown="True" "Data transfer method" {
      tunnel: w339 -> [w372 w375]
      tunnel: [w371 w373] -> w338
      tunnel: "Downsample" -> [w370 _]
      tunnel: w333 -> [_ w374]
      frame False {
        n161 = Divide(x=w372, y=w370) -> (x/y=w371:dbl)
      }
      frame True {
        n162 = Divide(x=w375, y=w374) -> (x/y=w373:dbl)
      }
    }
    n163 = xnode "Invoke Method"("FPGA VI Reference In"=w357, "error in"=w356, "Number of Elements"=w359) -> ("FPGA VI Reference Out"=w368:refnum<k20>, "error out"=w355:errorcluster, "Data"=w332:i16[])  [unwired: 1 in, 1 out]
    n164 = call "Scale Acquired Data + Separate Timeshare Data.vi"("range (V)"=w351, "Sample Rate"=w338, "Number of Bits"=i16 16, "Data In"=w332) -> ("Data"=→"AI":waveform(dbl)[])  [unwired: 4 in, 3 out]
    n165 = Index Array(array=w332, index=3) -> ()  [unwired: 1 out]
    n166 = in-place {
      in-place-border: [w377] -> w365
      in-place-border: w355 -> [w379]
      n167 = in-place-dvr #7(w364) -> (w378:bool, w376:errorcluster)
      n168 = Compound Arithmetic op=OR(w379, w378, w376) -> (w377:bool)
      n169 = in-place-dvr #7(w377) -> ()  [unwired: 2 out]
    }
    n170 = Wait (ms)(milliseconds to wait=u32 100) -> ()  [unwired: 1 out]
  }
  n171 = Merge Errors(w9, w8) -> (w11:errorcluster)
  n172 = xnode "Read/Write Control"("FPGA VI Reference In"=w17, "error in"=w11, "stream.request state 2"=3) -> ("FPGA VI Reference Out"=w14:refnum<k20>, "error out"=w16:errorcluster)
  n173 = xnode "Close FPGA VI Reference"("FPGA VI Reference In"=w14, "error in"=w16) -> ("error out"=w24:errorcluster)
  n174 = call <vilib>:"Simple Error Handler.vi"("error in (no error)"=w24) -> ("error out"=→"Error Out":errorcluster)  [unwired: 4 in, 4 out]
